vi "三角形面积.vi"(10 "y":dbl, 11 "x":dbl) -> (3 "result":dbl)   [LabVIEW 2013]
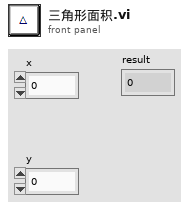
[diagram p1: front panel]
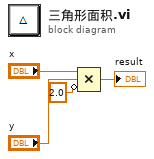
[diagram p0: block diagram]
diagram:
  n1 = Compound Arithmetic op=MULTIPLY("x", "y", invert 2.0 ("值")) -> (→"result":dbl)
